vi "Card1 Suit.vi"(6 "SS Path":path, 7 "error in (no error)":errorcluster, 10 "ROI 1st Card":T1) -> (0 "error out":errorcluster, 3 "Suit Card 1":T2)   [LabVIEW 2015]
uses:
  Suit Enum.ctl
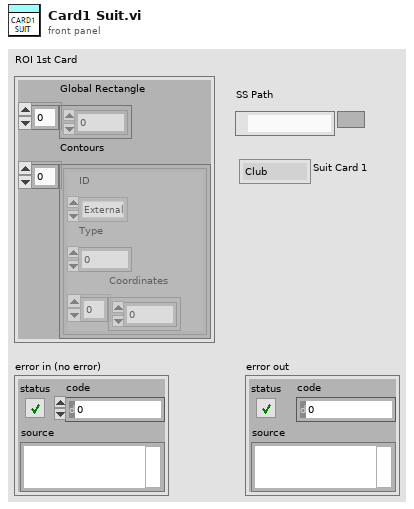
[diagram p1: front panel]
types:
  T1 = cluster{"Global Rectangle":i32[], "Contours":cluster{"ID":enum32{"External", "Internal"}, "Type":u32, "Coordinates":i32[]}[]}
  T2 = typedef "Suit Enum.ctl" = enum16{"Club", "Diamond", "Heart", "Spade", "Unknown", "Stop"}
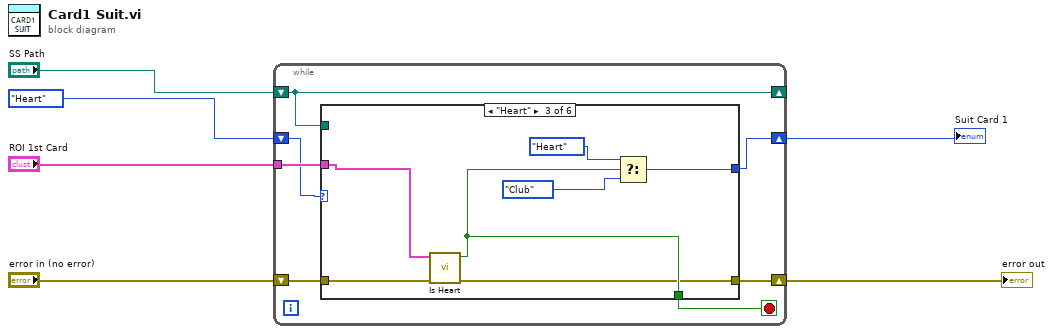
[diagram p0: block diagram]
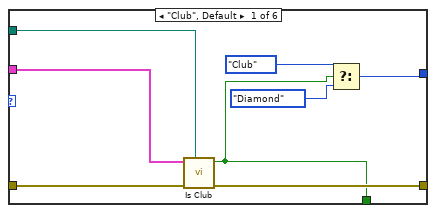
[diagram p2: hidden frame]
diagram:
  n1 = while {
    tunnel: "ROI 1st Card" -> [w13]
    shift-right: [w9] -> w4
    shift-left: "error in (no error)" -> [w12]
    shift-right: [w11] -> _
    shift-left: "SS Path" -> [w11]
    shift-right: [w7] -> w2
    shift-left: Suit_Enum."Heart" ("Suit Card 1") -> [w8]
    stop <- w10 stop-if-true
    n2 = case shown="\"Heart\"" w8 {
      tunnel: w13 -> [w19 _ w29 _ _ _]
      tunnel: w12 -> [w20 w22 w26 _ _ _]
      tunnel: w11 -> [w18 _ _ _ _ _]
      tunnel: [w17 _ w28 _ _ _] -> w7
      tunnel: [w16 _ w27 _ _ _] -> w10
      tunnel: [w21 w22 w25 _ _ _] -> w9
      frame "Club", Default {
        n3 = call "Is Club.vi"("File Path"=w18, "error in"=w20, "ROI Descriptor (Club Match)"=w19) -> ("error out"=w21:errorcluster, "IS Club"=w16:bool)  [unwired: 6 in, 1 out]
        n4 = Select(t=Suit_Enum."Club" ("Suit Card 1"), s=w16, f=Suit_Enum."Diamond" ("Suit Card 1")) -> (s? t:f=w17:T2)
      }
      frame "Diamond" {
      }
      frame "Heart" {
        n5 = call "Is Heart.vi"("error in"=w26, "ROI Descriptor (Heart Match)"=w29) -> ("error out"=w25:errorcluster, "Found Heart"=w27:bool)  [unwired: 7 in, 1 out]
        n6 = Select(t=Suit_Enum."Heart" ("Suit Card 1"), s=w27, f=Suit_Enum."Club" ("Suit Card 1")) -> (s? t:f=w28:T2)
      }
      frame "Spade" {
      }
      frame "Unknown" {
      }
      frame "Stop" {
      }
    }
  }
  "Suit Card 1" <- w2
  "error out" <- w4
